vi "Create Plugin Interface Pool.vi"(7 "FIFO Options":T1, 8 "error in (no error)":errorcluster, 10 "interface fifo depths (10)":u32=10, 11 "number of interfaces":u32) -> (0 "error out":errorcluster, 3 "Plugin Thread Pool out":refnum<class "Plugin Interface Pool.lvclass">)   [LabVIEW 2017, in "DSF Core.lvlib" / "Plugin Interface Pool.lvclass"]
uses:
  Plugin Interface Pool.lvclass
  C:/Git/DSF/Data Sharing Framework Core/Classes/Thread Pool/Pool.lvclass
  Typedefs/DSF FIFO Options.ctl
  Pool.lvclass/Pool.ctl
  Plugin Interface Pool.lvclass/Plugin Interface Pool.ctl
  Pool.lvclass
  Interfaces/Plugin/Plugin Interface.lvclass
  DSF Core.lvlib
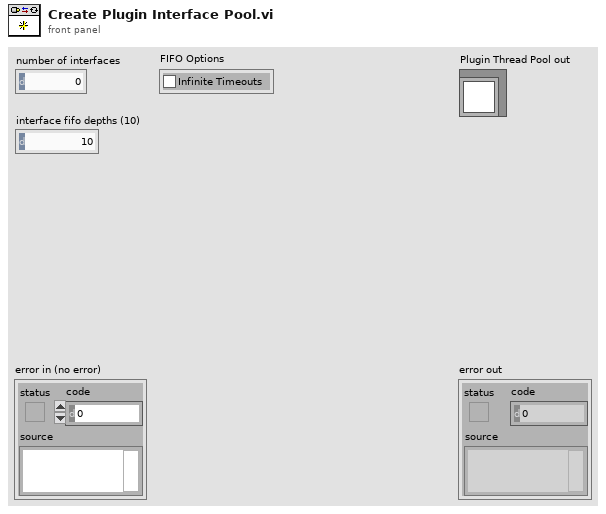
[diagram p1: front panel]
types:
  T1 = typedef "DSF Core.lvlib/DSF FIFO Options.ctl" = cluster{"Infinite Timeouts":bool}
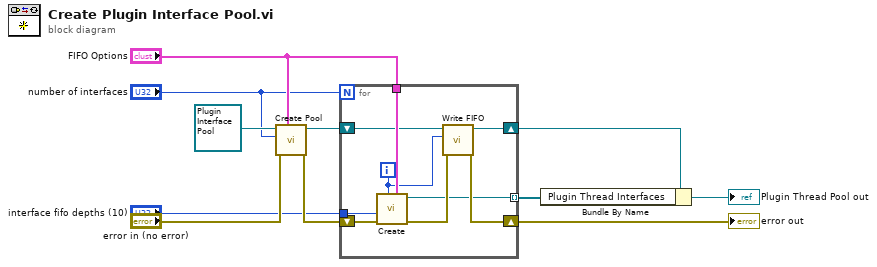
[diagram p0: block diagram]
diagram:
  n1 = call "Create Pool.vi"("FIFO Options"="FIFO Options", "error in (no error)"="error in (no error)", "number of elements"="number of interfaces", "Pool type"=refnum<class "Plugin Interface Pool.lvclass"> refnum ("Plugin Thread Pool in")) -> ("error out"=w7:errorcluster, "Pool"=w4:refnum<class "Plugin Interface Pool.lvclass">)  [unwired: 6 in]
  n2 = for {
    N: "number of interfaces" -> [_]
    tunnel: [w12] -> w9 mode=indexing
    shift-right: [w15] -> w10
    shift-left: w7 -> [w20]
    tunnel: "FIFO Options" -> [w19]
    tunnel: "interface fifo depths (10)" -> [w18]
    shift-right: [w14] -> w3
    shift-left: w4 -> [w17]
    i -> [w13]
    n3 = call "Create.vi"("FIFO Options"=w19, "id (0)"=w13, "error in (no error)"=w20, "fifo depths (10)"=w18) -> ("error out"=w16:errorcluster, "Plugin Interface"=w12:refnum<class "Plugin Interface.lvclass">)  [unwired: 6 in]
    n4 = call "Write FIFO.vi"("error in (no error)"=w16, "element"=w13, "Pool in"=w17) -> ("error out"=w15:errorcluster, "Pool out"=w14:refnum<class "Plugin Interface Pool.lvclass">)  [unwired: 6 in, 1 out]
  }
  "error out" <- w10
  n5 = Bundle By Name(cluster=w3, "Plugin Thread Interfaces"=w9) -> (→"Plugin Thread Pool out":refnum<class "Plugin Interface Pool.lvclass">)
